vi "Send_Notifier.vi"(7 "Device Number":T1, 9 "Stream Type":T2, 11 "navX Action":T3) -> ()   [LabVIEW 2016]
uses:
  TypeDefs/Z900_navX_ActionTypeDef.ctl
  navX Library v2.lvlib
  TypeDefs/Z900_navX_SerialStreamTypeDef.ctl
  TypeDefs/FRIC_navX_DeviceNumbersTypeDef.ctl
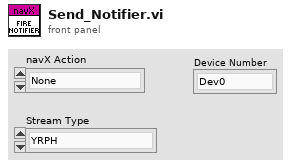
[diagram p1: front panel]
types:
  T1 = typedef "FRIC_navX_DeviceNumbersTypeDef.ctl" = enum16{"Dev0", "Dev1", "Dev2", "Dev3"}
  T2 = typedef "navX Library v2.lvlib/Z900_navX_SerialStreamTypeDef.ctl" = enum16{"YRPH", "Quaterinons", "Gyro/Raw", "AHRS", "AHRSAndPositioning"}
  T3 = typedef "navX Library v2.lvlib/Z900_navX_ActionTypeDef.ctl" = enum16{"None", "Halt", "Update Serial Protocol", "Zero-Yaw", "Zero-Displacement", "Zero-Velocity"}
  T4 = typedef "navX Library v2.lvlib/Z900_navX_NotifyPacketTypeDef.ctl" = cluster{"navX Action":T3, "Data":variant}
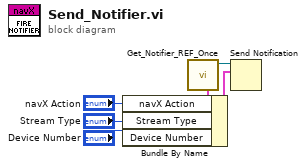
[diagram p0: block diagram]
diagram:
  n1 = call "Get_Notifier_REF_Once.vi"() -> ("notifier ref out"=w6:refnum<notifier>, "notification"=w5:T4)  [unwired: 10 in]
  n2 = Bundle By Name(cluster=w5, "navX Action"="navX Action", "Stream Type"="Stream Type", "Device Number"="Device Number") -> (w4:T4)
  n3 = Send Notification(notification=w4, notifier=w6) -> ()  [unwired: 1 in, 2 out]
